vi "Read Data From LabVIEW INI.vi"(8 "error in":errorcluster, 10 "DNL_Font":refnum<vi>, 11 "IE VI Ref":refnum<vi>) -> (0 "error out":errorcluster, 3 "INI Data":T1={"Show Terminals?"=FALSE, "Text"={"Font"="Small Fonts", "Alignment"=0, "Size"=9}, "3rd party Templates"={"Store 3rd party Templates?"=TRUE, "Folder Name"="3rd party"}, "Merge user layers on commit"=TRUE, "Body Text"={"Line 1 text"="", "Line 2 text"="", "Line 3 text"="", "Line 4 text"="", "Line 1 color"=0, "Line 2 color"=0, "Line 3 color"=0, "Line 4 color"=0, "Body Text Spec"={"Font"="", "Alignment"=0, "Size"=3}, "Center text vertically"=FALSE, "Capitalize Text"=FALSE}, "Fill Color"=16711680, "Edge Color"=0, "Tab"=0, "Tool"=enum."Ellipse", "Disable Layers?"=FALSE} {"Body Text"."Body Text Spec"."Alignment" items=["left", "center", "right"]; "Text"."Alignment" items=["left", "center", "right"]})   [LabVIEW 2020, in "lv_icon.lvlib"]
uses:
  vi.lib/LabVIEW Icon API/lv_icon/lv_icon.lvlib
  <resource>/dialog/lvconfig.llb/LV Config Read String.vi
  <resource>/dialog/lvconfig.llb/LV Config Read Color.vi
  <resource>/dialog/lvconfig.llb/LV Config Read Boolean.vi
  vi.lib/LabVIEW Icon API/lv_icon/Controls/Font.ctl
  vi.lib/LabVIEW Icon API/lv_icon/Controls/Alignment.ctl
  Controls/Font Size.ctl
  vi.lib/LabVIEW Icon API/lv_icon/Controls/BodyText.ctl
  vi.lib/LabVIEW Icon API/lv_icon/Controls/IEColor.ctl
  Controls/Tools.ctl
  INI Data.ctl
  b61c55f6-cb00-4273-a894-d9276d43ab4a.vi
  Controls/Circle.ctl
  Controls/Dropper.ctl
  Controls/FCircle.ctl
  Controls/Fill.ctl
  Controls/FRect.ctl
  Controls/Line.ctl
  Controls/Move.ctl
  Controls/Pen.ctl
  Controls/IERect.ctl
  Controls/Rubber.ctl
  Controls/Selection.ctl
  Controls/Text.ctl
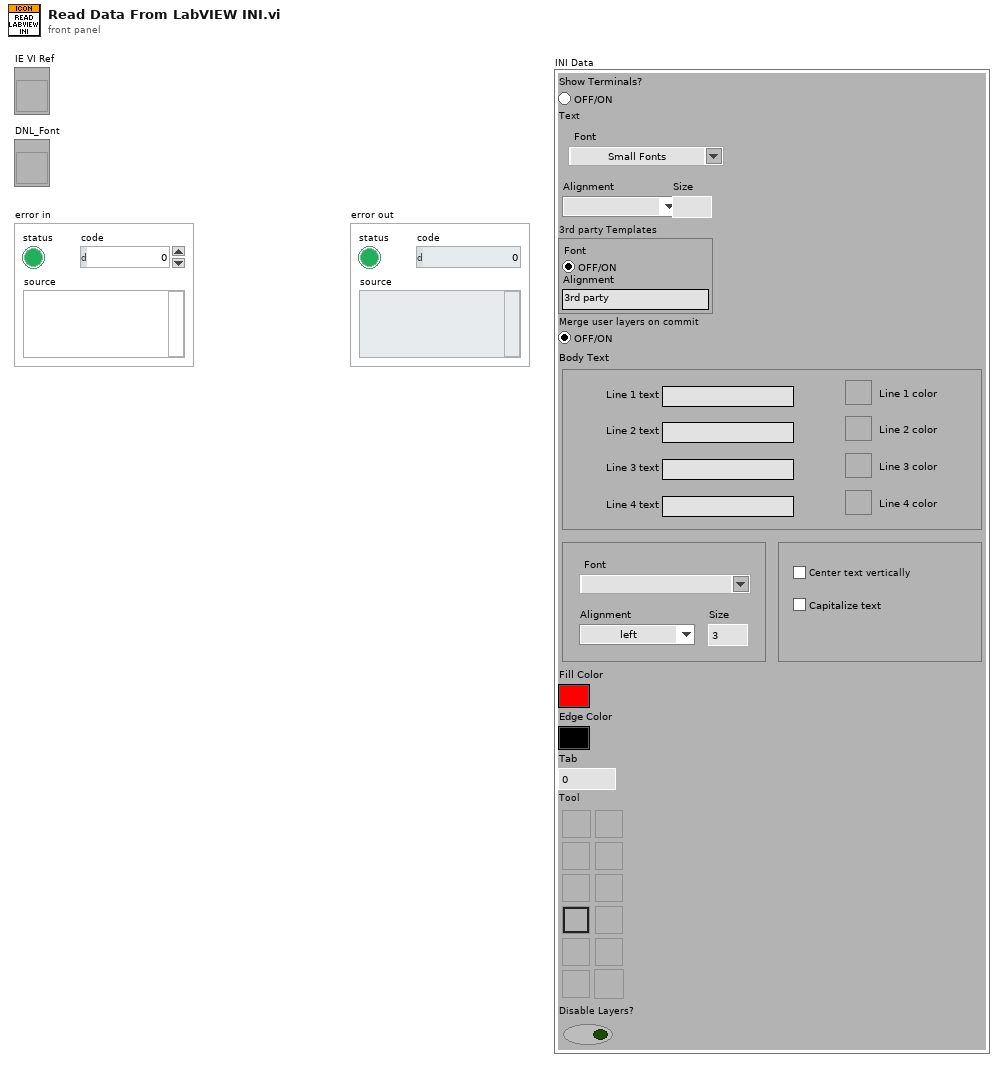
[diagram p1: front panel]
types:
  T1 = typedef "lv_icon.lvlib/INI Data.ctl" = cluster{"Show Terminals?":bool, "Text":cluster{"Font":T2, "Alignment":T3, "Size":T4}, "3rd party Templates":cluster{"Store 3rd party Templates?":bool, "Folder Name":string}, "Merge user layers on commit":bool, "Body Text":T5, "Fill Color":T6, "Edge Color":T6, "Tab":u16, "Tool":T7, "Disable Layers?":bool}
  T2 = typedef "Font.ctl" = string
  T3 = typedef "Alignment.ctl" = u16
  T4 = typedef "Font Size.ctl" = u8
  T5 = typedef "BodyText.ctl" = cluster{"Line 1 text":string, "Line 2 text":string, "Line 3 text":string, "Line 4 text":string, "Line 1 color":u32, "Line 2 color":u32, "Line 3 color":u32, "Line 4 color":u32, "Body Text Spec":cluster{"Font":T2, "Alignment":T3, "Size":u8}, "Center text vertically":bool, "Capitalize Text":bool}
  T6 = typedef "IEColor.ctl" = u32
  T7 = typedef "Tools.ctl" = enum32{"Pencil", "Line", "Dropper", "Fill", "Rectangle", "Filled Rectangle", "Ellipse", "Filled Ellipse", "Eraser", "Text", "Select", "Move"}
  T8 = enum16{"Show Terminals?", "Text Font", "Text Alignment", "Text Size", "Store 3rd Party Templates?", "Templates Folder Name", "Merge User Layers on Commit", "Body Text Colors", "Body Text Spec", "Body Text Options", "Fill Color", "Edge Color", "Tab", "Tool", "Disable Layers?", "Position", "FirstCall"}
  T9 = enum16{"Show Terminals?", "Text Font", "Text Alignment", "Text Size", "Store 3rd Party Templates?", "Templates Folder Name", "Merge User Layers on Commit", "Body Text Colors", "Body Text Spec", "Body Text Options", "Fill Color", "Edge Color", "Tab", "Tool", "Disable Layers?", "Position", "FirstCall"}[]
  T10 = typedef "LVRectTypeDef.ctl" = cluster{"Left":i16, "Top":i16, "Right":i16, "Bottom":i16}
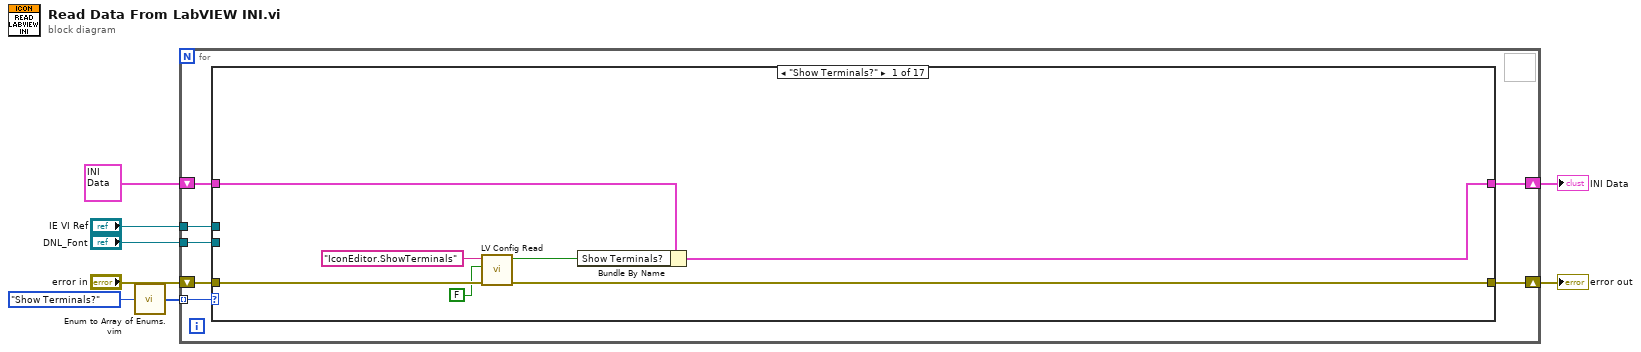
[diagram p0: block diagram]
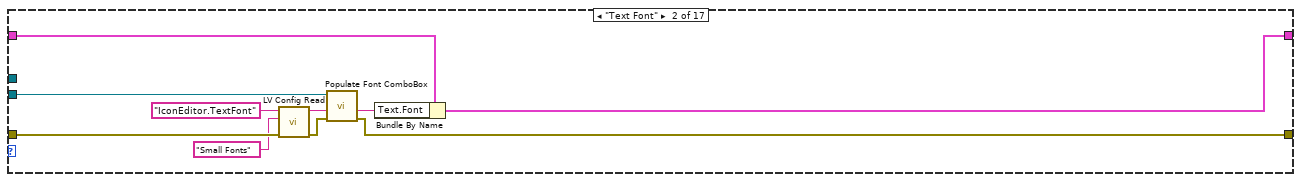
[diagram p2: hidden frame]
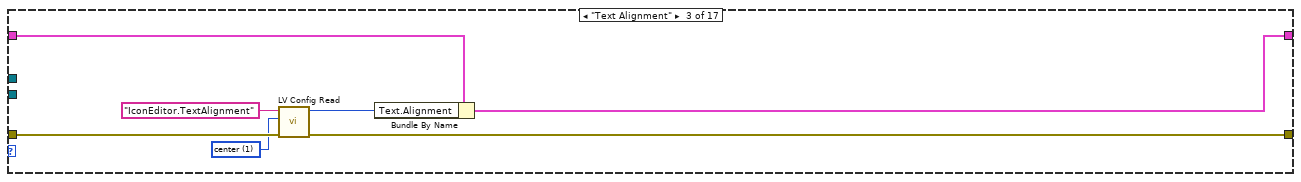
[diagram p3: hidden frame]
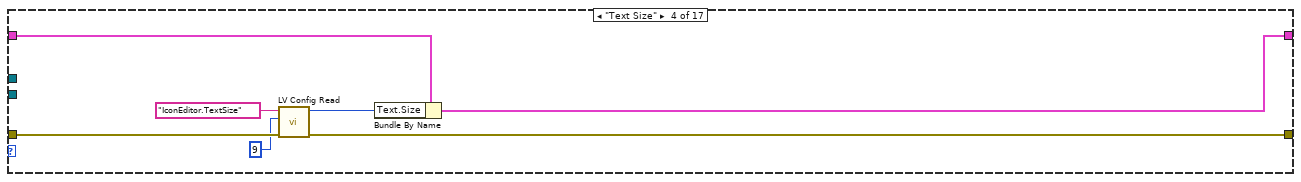
[diagram p4: hidden frame]
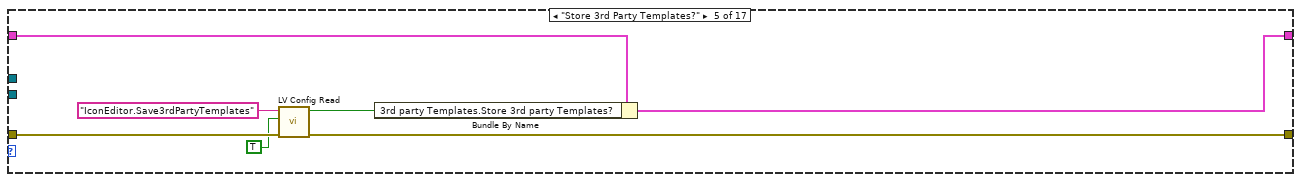
[diagram p5: hidden frame]
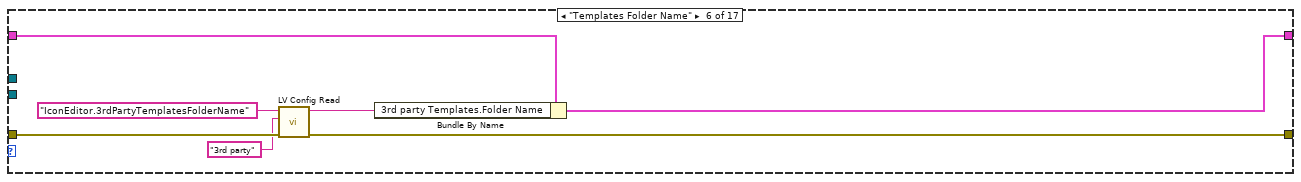
[diagram p6: hidden frame]
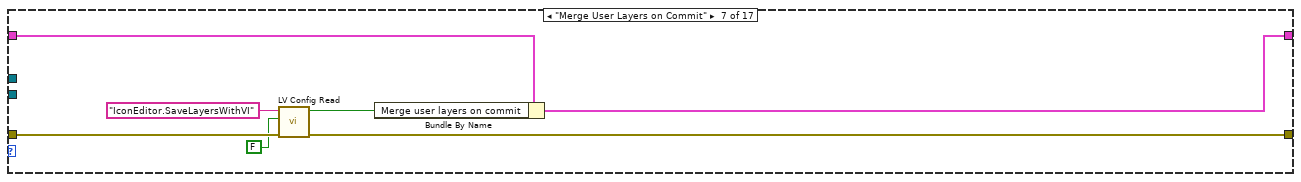
[diagram p7: hidden frame]
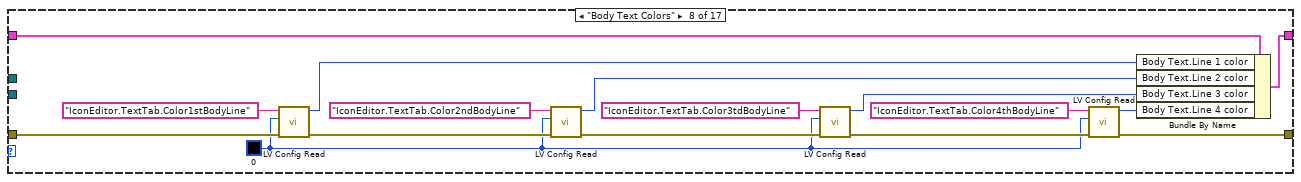
[diagram p8: hidden frame]
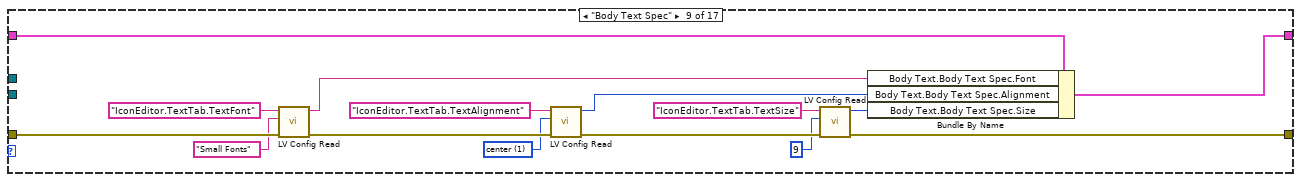
[diagram p9: hidden frame]
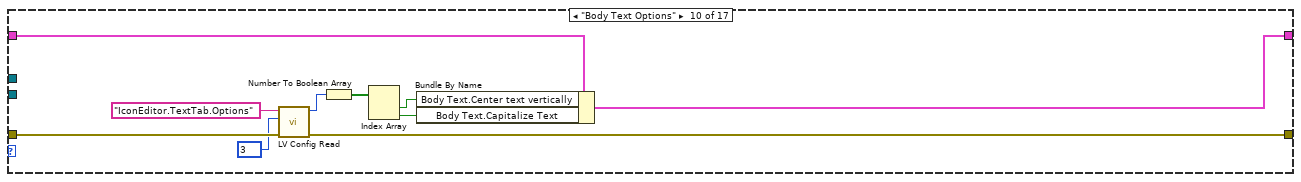
[diagram p10: hidden frame]
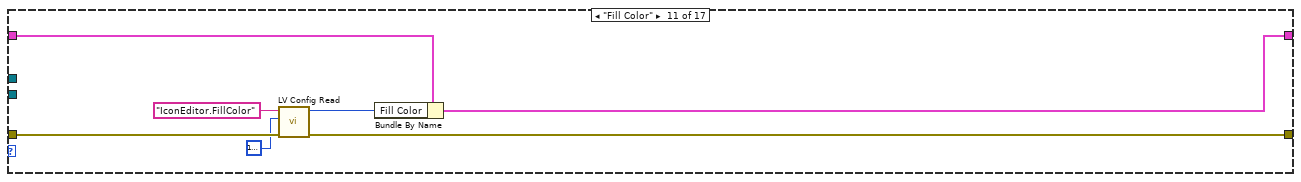
[diagram p11: hidden frame]
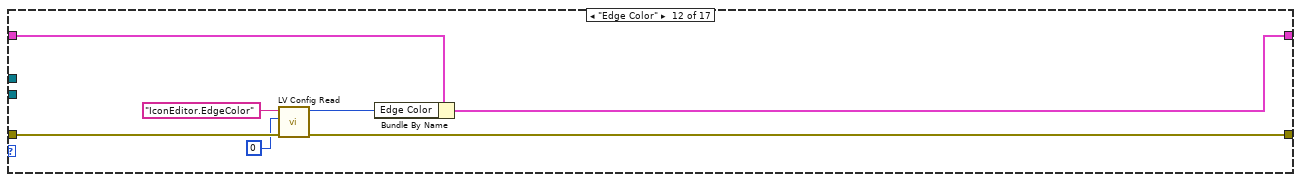
[diagram p12: hidden frame]
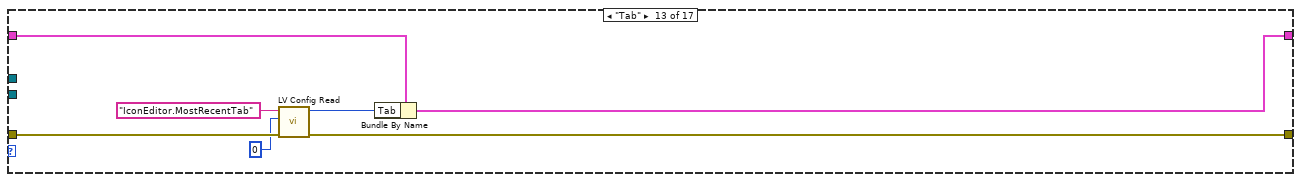
[diagram p13: hidden frame]
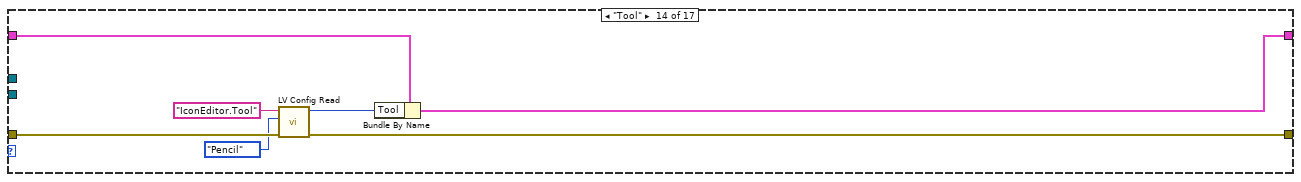
[diagram p14: hidden frame]
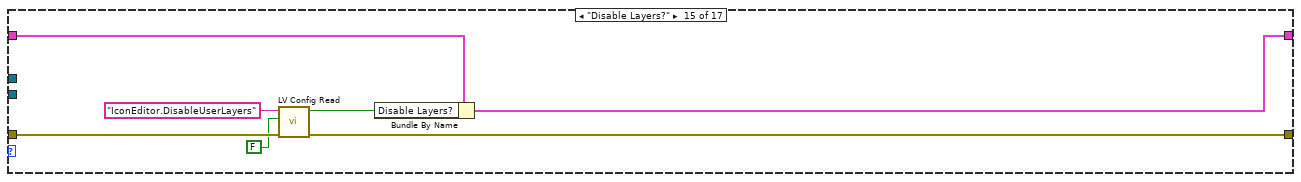
[diagram p15: hidden frame]
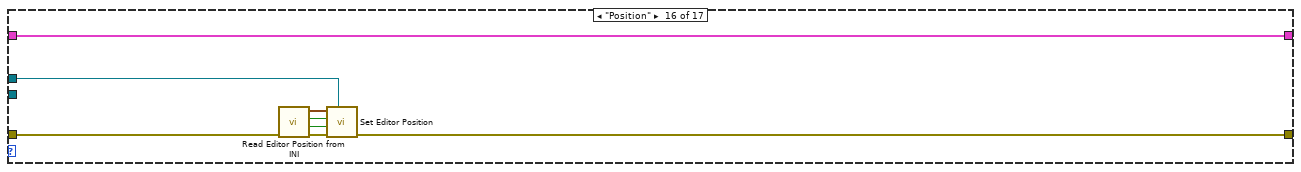
[diagram p16: hidden frame]
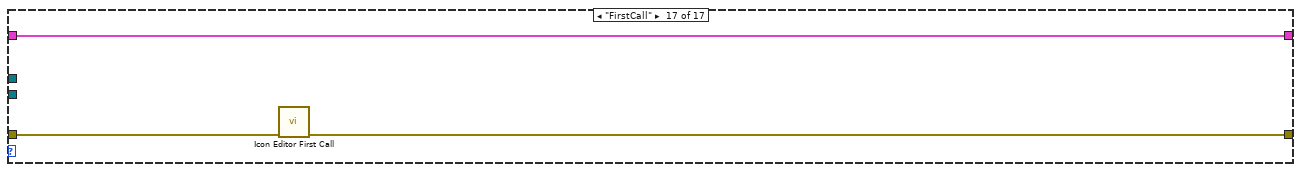
[diagram p17: hidden frame]
diagram:
  n1 = call "Enum to Array of Enums.vim"("enum"=T8."Show Terminals?") -> ("array of enums"=w4:T9)
  n2 = for {
    shift-right: [w11] -> w1
    shift-left: T1 {"Show Terminals?"=FALSE, "Text"={"Font"="Small Fonts", "Alignment"=1, "Size"=9}, "3rd party Templates"={"Store 3rd party Templates?"=TRUE, "Folder Name"="3rd party"}, "Merge user layers on commit"=FALSE, "Body Text"={"Line 1 text"="", "Line 2 text"="", "Line 3 text"="", "Line 4 text"="", "Line 1 color"=0, "Line 2 color"=0, "Line 3 color"=0, "Line 4 color"=0, "Body Text Spec"={"Font"="Small Fonts", "Alignment"=1, "Size"=9}, "Center text vertically"=TRUE, "Capitalize Text"=TRUE}, "Fill Color"=16711680, "Edge Color"=0, "Tab"=0, "Tool"=enum."Pencil", "Disable Layers?"=FALSE} ("INI Data") -> [w12]
    tunnel: w4 -> [w13] mode=indexing
    shift-right: [w14] -> w7
    shift-left: "error in" -> [w15]
    tunnel: "DNL_Font" -> [w10]
    tunnel: "IE VI Ref" -> [w9]
    n3 = case shown="\"Show Terminals?\"" w13 {
      tunnel: w12 -> [w20 w29 w37 w44 w51 w58 w65 w78 w94 w106 w113 w120 w127 w134 w141 w148 w152]
      tunnel: w15 -> [w22 w32 w39 w46 w53 w60 w67 w83 w98 w108 w115 w122 w129 w136 w143 w150 w154]
      tunnel: [w17 w27 w34 w41 w48 w55 w62 w75 w91 w104 w110 w117 w124 w131 w138 w148 w152] -> w11
      tunnel: [w21 w30 w38 w45 w52 w59 w66 w79 w95 w107 w114 w121 w128 w135 w142 w151 w153] -> w14
      tunnel: w10 -> [_ w26 _ _ _ _ _ _ _ _ _ _ _ _ _ _ _]
      tunnel: w9 -> [_ _ _ _ _ _ _ _ _ _ _ _ _ _ _ w147 _]
      frame "Show Terminals?" {
        n4 = call-poly <resource>:"LV Config Read.vi"("error in"=w22, "default value"=FALSE, "key"="IconEditor.ShowTerminals") -> ("error out"=w21:errorcluster, "value"=w18:bool)  [unwired: 3 out]
        n5 = Bundle By Name(cluster=w20, "Show Terminals?"=w18) -> (w17:T1)
      }
      frame "Text Font" {
        n6 = call-poly <resource>:"LV Config Read.vi"("error in"=w32, "default value"="Small Fonts", "key"="IconEditor.TextFont") -> ("error out"=w31:errorcluster, "value"=w25:string)  [unwired: 3 out]
        n7 = call "Populate Font ComboBox.vi"("error in"=w31, "Font in"=w25, "CmbBox Refnum"=w26) -> ("error out"=w30:errorcluster, "Font out"=w24:string)  [unwired: 7 out]
        n8 = Bundle By Name(cluster=w29, "Text.Font"=w24) -> (w27:T1)
      }
      frame "Text Alignment" {
        w33 = T3 1 items=["left", "center", "right"] ("Alignment")
        n9 = call-poly <resource>:"LV Config Read.vi"("error in"=w39, "default value"=w33, "key"="IconEditor.TextAlignment") -> ("error out"=w38:errorcluster, "value"=w35:u32)  [unwired: 3 out]
        n10 = Bundle By Name(cluster=w37, "Text.Alignment"=w35) -> (w34:T1)
      }
      frame "Text Size" {
        n11 = call-poly <resource>:"LV Config Read.vi"("error in"=w46, "default value"=T4 9 ("Size"), "key"="IconEditor.TextSize") -> ("error out"=w45:errorcluster, "value"=w42:u32)  [unwired: 2 in, 1 out]
        n12 = Bundle By Name(cluster=w44, "Text.Size"=w42) -> (w41:T1)
      }
      frame "Store 3rd Party Templates?" {
        n13 = call-poly <resource>:"LV Config Read.vi"("error in"=w53, "default value"=TRUE, "key"="IconEditor.Save3rdPartyTemplates") -> ("error out"=w52:errorcluster, "value"=w49:bool)  [unwired: 3 out]
        n14 = Bundle By Name(cluster=w51, "3rd party Templates.Store 3rd party Templates?"=w49) -> (w48:T1)
      }
      frame "Templates Folder Name" {
        n15 = call-poly <resource>:"LV Config Read.vi"("error in"=w60, "default value"="3rd party", "key"="IconEditor.3rdPartyTemplatesFolderName") -> ("error out"=w59:errorcluster, "value"=w56:string)  [unwired: 3 out]
        n16 = Bundle By Name(cluster=w58, "3rd party Templates.Folder Name"=w56) -> (w55:T1)
      }
      frame "Merge User Layers on Commit" {
        n17 = call-poly <resource>:"LV Config Read.vi"("error in"=w67, "default value"=FALSE, "key"="IconEditor.SaveLayersWithVI") -> ("error out"=w66:errorcluster, "value"=w63:bool)  [unwired: 3 out]
        n18 = Bundle By Name(cluster=w65, "Merge user layers on commit"=w63) -> (w62:T1)
      }
      frame "Body Text Colors" {
        w68 = u32 0 ("Line 1 color")
        n19 = call-poly <resource>:"LV Config Read.vi"("error in"=w83, "default value"=w68, "key"="IconEditor.TextTab.Color1stBodyLine") -> ("error out"=w82:errorcluster, "value"=w76:u32)  [unwired: 3 out]
        n20 = call-poly <resource>:"LV Config Read.vi"("error in"=w82, "default value"=w68, "key"="IconEditor.TextTab.Color2ndBodyLine") -> ("error out"=w81:errorcluster, "value"=w69:u32)  [unwired: 3 out]
        n21 = call-poly <resource>:"LV Config Read.vi"("error in"=w81, "default value"=w68, "key"="IconEditor.TextTab.Color3tdBodyLine") -> ("error out"=w80:errorcluster, "value"=w70:u32)  [unwired: 3 out]
        n22 = call-poly <resource>:"LV Config Read.vi"("error in"=w80, "default value"=w68, "key"="IconEditor.TextTab.Color4thBodyLine") -> ("error out"=w79:errorcluster, "value"=w71:u32)  [unwired: 3 out]
        n23 = Bundle By Name(cluster=w78, "Body Text.Line 1 color"=w76, "Body Text.Line 2 color"=w69, "Body Text.Line 3 color"=w70, "Body Text.Line 4 color"=w71) -> (w75:T1)
      }
      frame "Body Text Spec" {
        w85 = T3 1 items=["left", "center", "right"] ("Alignment")
        n24 = call-poly <resource>:"LV Config Read.vi"("error in"=w98, "default value"="Small Fonts", "key"="IconEditor.TextTab.TextFont") -> ("error out"=w97:errorcluster, "value"=w92:string)  [unwired: 3 out]
        n25 = call-poly <resource>:"LV Config Read.vi"("error in"=w97, "default value"=w85, "key"="IconEditor.TextTab.TextAlignment") -> ("error out"=w96:errorcluster, "value"=w87:u32)  [unwired: 3 out]
        n26 = call-poly <resource>:"LV Config Read.vi"("error in"=w96, "default value"=u8 9 ("Size"), "key"="IconEditor.TextTab.TextSize") -> ("error out"=w95:errorcluster, "value"=w88:u32)  [unwired: 3 out]
        n27 = Bundle By Name(cluster=w94, "Body Text.Body Text Spec.Font"=w92, "Body Text.Body Text Spec.Alignment"=w87, "Body Text.Body Text Spec.Size"=w88) -> (w91:T1)
      }
      frame "Body Text Options" {
        n28 = call-poly <resource>:"LV Config Read.vi"("error in"=w108, "default value"=u32 3, "key"="IconEditor.TextTab.Options") -> ("error out"=w107:errorcluster, "value"=w102:u32)  [unwired: 3 out]
        n29 = Number To Boolean Array(number=w102) -> (Boolean array=w103:bool[])
        n30 = Index Array(array=w103) -> (element #1=w101:bool, element #2=w100:bool)  [unwired: 2 in]
        n31 = Bundle By Name(cluster=w106, "Body Text.Center text vertically"=w101, "Body Text.Capitalize Text"=w100) -> (w104:T1)
      }
      frame "Fill Color" {
        n32 = call-poly <resource>:"LV Config Read.vi"("error in"=w115, "default value"=T6 16711680 ("Fill Color"), "key"="IconEditor.FillColor") -> ("error out"=w114:errorcluster, "value"=w111:u32)  [unwired: 3 out]
        n33 = Bundle By Name(cluster=w113, "Fill Color"=w111) -> (w110:T1)
      }
      frame "Edge Color" {
        n34 = call-poly <resource>:"LV Config Read.vi"("error in"=w122, "default value"=T6 0 ("Edge Color"), "key"="IconEditor.EdgeColor") -> ("error out"=w121:errorcluster, "value"=w118:u32)  [unwired: 3 out]
        n35 = Bundle By Name(cluster=w120, "Edge Color"=w118) -> (w117:T1)
      }
      frame "Tab" {
        n36 = call-poly <resource>:"LV Config Read.vi"("error in"=w129, "default value"=u16 0 ("Tab"), "key"="IconEditor.MostRecentTab") -> ("error out"=w128:errorcluster, "value"=w125:u32)  [unwired: 3 out]
        n37 = Bundle By Name(cluster=w127, "Tab"=w125) -> (w124:T1)
      }
      frame "Tool" {
        n38 = call-poly <resource>:"LV Config Read.vi"("error in"=w136, "default value"=Tools."Pencil" ("Tool"), "key"="IconEditor.Tool") -> ("error out"=w135:errorcluster, "value"=w132:u32)  [unwired: 3 out]
        n39 = Bundle By Name(cluster=w134, "Tool"=w132) -> (w131:T1)
      }
      frame "Disable Layers?" {
        n40 = call-poly <resource>:"LV Config Read.vi"("error in"=w143, "default value"=FALSE, "key"="IconEditor.DisableUserLayers") -> ("error out"=w142:errorcluster, "value"=w139:bool)  [unwired: 3 out]
        n41 = Bundle By Name(cluster=w141, "Disable Layers?"=w139) -> (w138:T1)
      }
      frame "Position" {
        n42 = call "Read Editor Position from INI.vi"("error in"=w150) -> ("error out"=w149:errorcluster, "Use Size"=w144:bool, "Bounds Valid"=w145:bool, "Window Bounds"=w146:T10)  [unwired: 7 in]
        n43 = call "Set Editor Position.vi"("IE VI Ref"=w147, "error in"=w149, "Use Size"=w144, "Bounds Vaid"=w145, "Window Bounds"=w146) -> ("error out"=w151:errorcluster)  [unwired: 6 in]
      }
      frame "FirstCall" {
        n44 = call "Icon Editor First Call.vi"("error in (no error)"=w154) -> ("error out"=w153:errorcluster)  [unwired: 10 out]
      }
    }
  }
  "INI Data" <- w1
  "error out" <- w7
